vi "hist11.vi"(3 "Y":i16[](array[numeric])) -> (0 "values":i16[](array[numeric]), 1 "q":i32[](array[numeric]))   [LabVIEW 2010]
panel:
  # "Вычисление точной гистограммы. Подсчитывается каждое имеющееся значение отдельно."
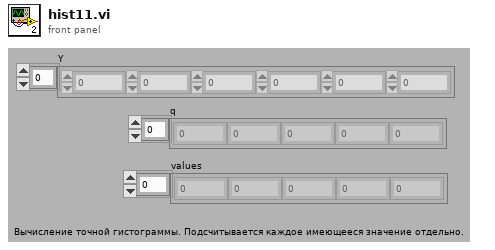
[diagram p1: front panel]
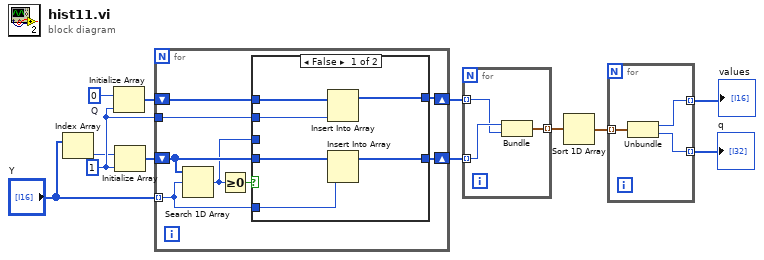
[diagram p0: block diagram]
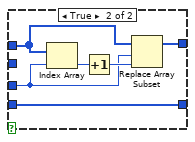
[diagram p2: hidden frame]
diagram:
  w11 = 0  # Q
  w9 = 1 ("dimension size")
  n1 = Index Array(array="Y") -> (element=w1:i16)  [unwired: 1 in]
  n2 = Initialize Array(w11, w9) -> (w10:i32[])
  n3 = Initialize Array(w1, w9) -> (w12:i16[])
  n4 = for {
    tunnel: "Y" -> [w17] mode=indexing
    shift-right: [w20] -> w7
    shift-left: w12 -> [w18]
    shift-right: [w16] -> w8
    shift-left: w10 -> [w15]
    tunnel: w9 -> [w13]
    n5 = Search 1D Array(1D array=w18, element=w17) -> (index of element=w14:i32)  [unwired: 1 in]
    n6 = Greater Or Equal To 0?(x=w14) -> (x >= 0?=w19:bool)
    n7 = case shown="False" w19 {
      tunnel: w18 -> [w26 w32]
      tunnel: [w25 w32] -> w20
      tunnel: w17 -> [w24 _]
      tunnel: [w23 w28] -> w16
      tunnel: w15 -> [w22 w29]
      tunnel: w14 -> [_ w27]
      tunnel: w13 -> [w21 _]
      frame False {
        n8 = Insert Into Array(array=w22, new element=w21) -> (w23:i32[])  [unwired: 1 in]
        n9 = Insert Into Array(array=w26, new element=w24) -> (w25:i16[])  [unwired: 1 in]
      }
      frame True {
        n10 = Index Array(array=w29, index=w27) -> (element=w31:i32)
        n11 = Increment(x=w31) -> (x+1=w30:i32)
        n12 = Replace Array Subset(array=w29, new element=w30, index=w27) -> (w28:i32[])
      }
    }
  }
  n13 = for {
    tunnel: w8 -> [w34] mode=indexing
    tunnel: w7 -> [w35] mode=indexing
    tunnel: [w33] -> w6 mode=indexing
    n14 = Bundle(w35, "Q"=w34) -> (w33:cluster{i16, "Q":i32})  [unwired: 1 in]
  }
  n15 = Sort 1D Array(array=w6) -> (sorted array=w5:cluster{i16, "Q":i32}[])
  n16 = for {
    tunnel: w5 -> [w38] mode=indexing
    tunnel: [w37] -> w4 mode=indexing
    tunnel: [w36] -> w3 mode=indexing
    n17 = Unbundle(w38) -> (w37:i16, "Q"=w36:i32)
  }
  "q" <- w3
  "values" <- w4
